vi "Digitizer_Trigger_Selection.vi"(3 "Error In":errorcluster, 4 "Channel Parameters In":T1, 5 "instrument handle in":refnum<k15>) -> (0 "error out":errorcluster, 1 "Channel Parameters Out":T1, 2 "instrument handle out":refnum<k15>)   [LabVIEW 2010]
uses:
  Typedef-Channel Parameters.ctl
  <instrlib>/niScope/Controls/niScope trigger slope.ctl
  <instrlib>/niScope/Controls/niScope trigger source.ctl
  <instrlib>/niScope/Controls/niScope export destinations.ctl
  <instrlib>/niScope/Controls/niScope exportable signals.ctl
  <instrlib>/niScope/Controls/niScope trigger source digital.ctl
  <instrlib>/niScope/Configure/Trigger/niScope Configure Trigger Edge.vi
  <instrlib>/niScope/Configure/Trigger/niScope Configure Trigger Digital.vi
  <instrlib>/niScope/Configure/Trigger/niScope Configure Trigger Immediate.vi
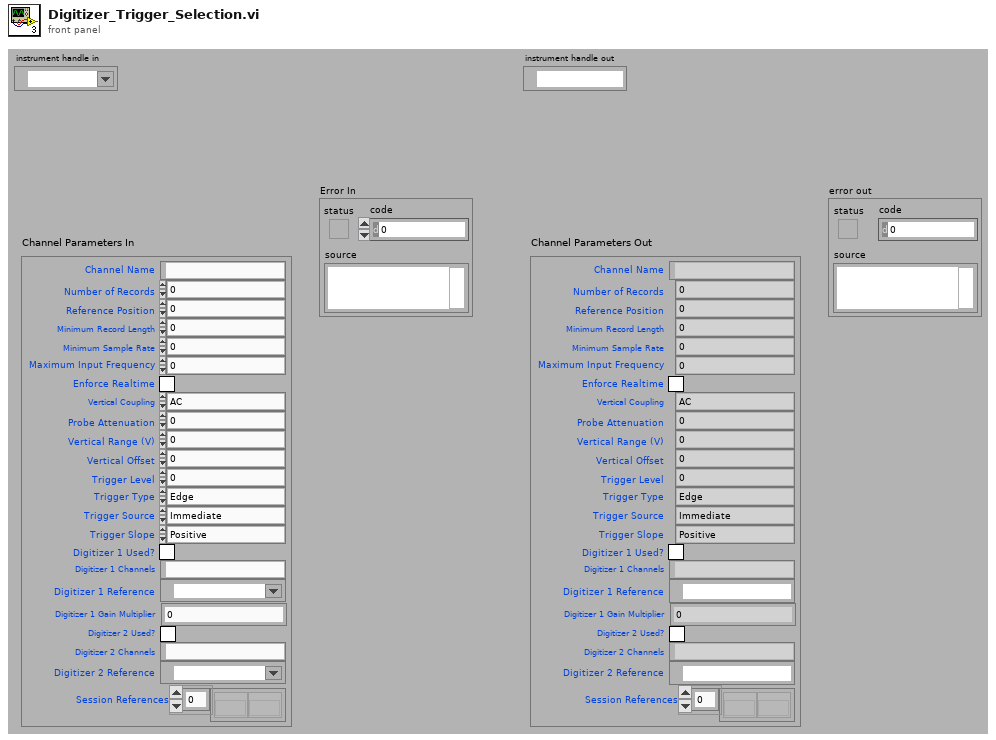
[diagram p1: front panel]
types:
  T1 = typedef "Typedef-Channel Parameters.ctl" = cluster{"Channel Name":string, "Number of Records":i32, "Reference Position":dbl, "Minimum Record Length":i32, "Minimum Sample Rate":dbl, "Maximum Input Frequency":dbl, "Enforce Realtime":bool, "Vertical Coupling":enum16{"AC", "DC", "Ground"}, "Probe Attenuation":dbl, "Vertical Range (V)":dbl, "Vertical Offset":dbl, "Trigger Level":dbl, "Trigger Type":enum16{"Edge", "Digital", "Immediate"}, "Trigger Source":enum16{"Immediate", "Channel 0", "Channel 1", "Channel 2", "Channel 3", "Channel 4", "Channel 5", "Channel 6", "Channel 7", "Extermal TRIG", "Software Trigger", "RTSI 0", "RTSI 1", "RTSI 2", "RTSI 3", "RTSI 4", "RTSI 5", "RTSI 6", "PF 0", "PF 1", "PF 2", "PXI Star Trigger"}, "Trigger Slope":enum16{"Positive", "Negative"}, "Digitizer 1 Used?":bool, "Digitizer 1 Channels":string, "Digitizer 1 Reference":refnum<k15>, "Digitizer 1 Gain Multiplier":dbl, "Digitizer 2 Used?":bool, "Digitizer 2 Channels":string, "Digitizer 2 Reference":refnum<k15>, "Session References":refnum<k20>[]}
  T2 = enum16{"Immediate", "Channel 0", "Channel 1", "Channel 2", "Channel 3", "Channel 4", "Channel 5", "Channel 6", "Channel 7", "Extermal TRIG", "Software Trigger", "RTSI 0", "RTSI 1", "RTSI 2", "RTSI 3", "RTSI 4", "RTSI 5", "RTSI 6", "PF 0", "PF 1", "PF 2", "PXI Star Trigger"}
  T3 = typedef "niScope trigger source.ctl" = string
  T4 = typedef "niScope export destinations.ctl" = string
  T5 = typedef "niScope trigger source digital.ctl" = string
  T6 = typedef "niScope trigger slope.ctl" = i32
  T7 = typedef "niScope exportable signals.ctl" = u16
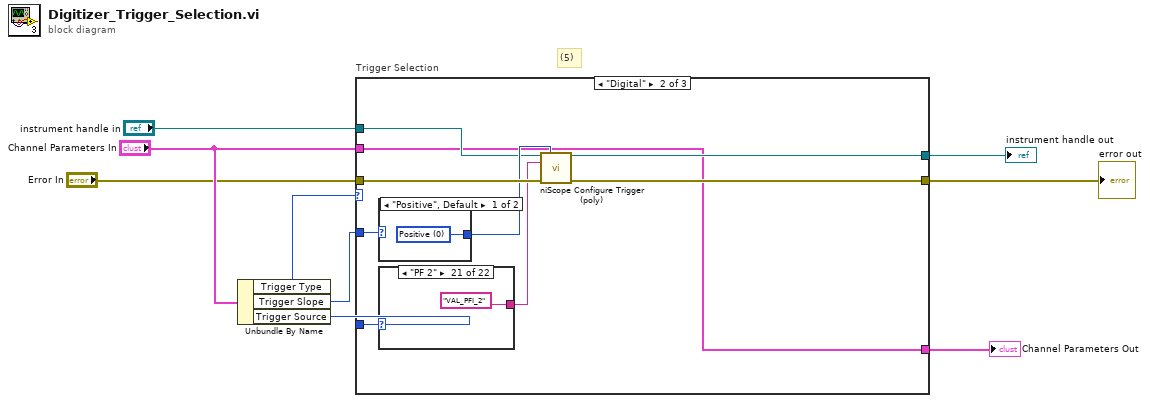
[diagram p0: block diagram]
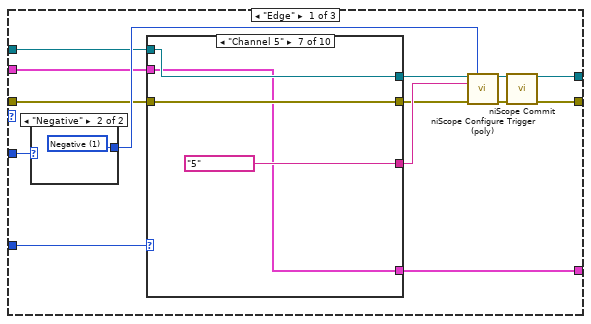
[diagram p2: hidden frame]
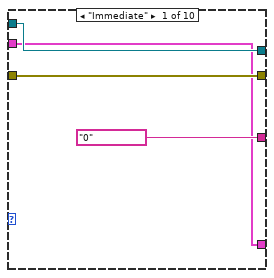
[diagram p3: hidden frame]
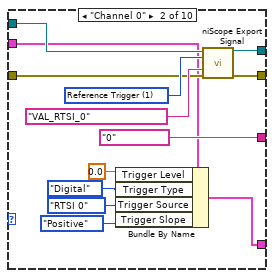
[diagram p4: hidden frame]
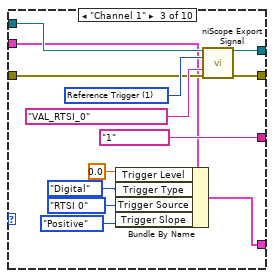
[diagram p5: hidden frame]
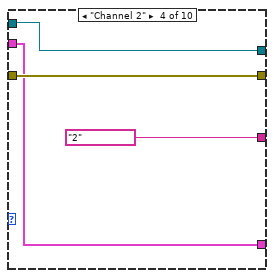
[diagram p6: hidden frame]
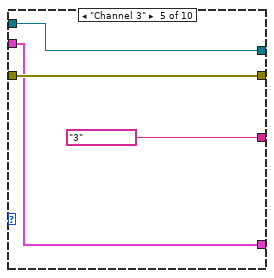
[diagram p7: hidden frame]
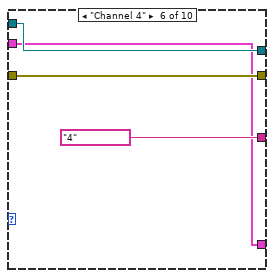
[diagram p8: hidden frame]
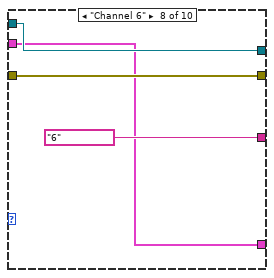
[diagram p9: hidden frame]
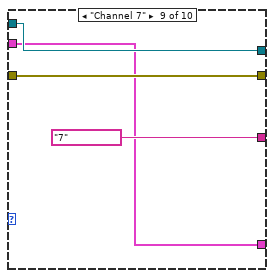
[diagram p10: hidden frame]
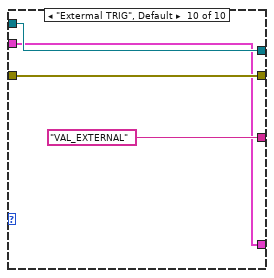
[diagram p11: hidden frame]
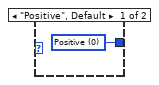
[diagram p12: hidden frame]
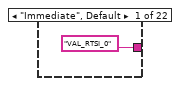
[diagram p13: hidden frame]
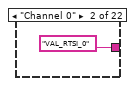
[diagram p14: hidden frame]
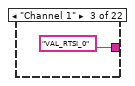
[diagram p15: hidden frame]
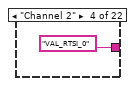
[diagram p16: hidden frame]
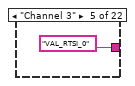
[diagram p17: hidden frame]
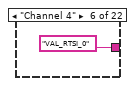
[diagram p18: hidden frame]
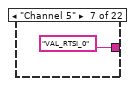
[diagram p19: hidden frame]
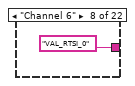
[diagram p20: hidden frame]
diagram:
  # "(5)"
  n1 = Unbundle By Name("Channel Parameters In") -> ("Trigger Type"=w1:enum16{"Edge", "Digital", "Immediate"}, "Trigger Slope"=w3:enum16{"Positive", "Negative"}, "Trigger Source"=w4:T2)
  n2 = case "Trigger Selection" shown="\"Digital\"" w1 {
    tunnel: "Error In" -> [w16 w92 w121]
    tunnel: [w18 w88 w120] -> w5
    tunnel: [w19 w89 w118] -> w9
    tunnel: w3 -> [w14 w87 _]
    tunnel: w4 -> [w13 w86 _]
    tunnel: [w12 w84 w117] -> w8
    tunnel: "Channel Parameters In" -> [w10 w84 w117]
    tunnel: "instrument handle in" -> [w11 w85 w119]
    frame "Edge" {
      n3 = case shown="\"Negative\"" w14 {
        tunnel: [w82 w83] -> w23
        frame "Positive", Default {
          w82 = T6 0 items=["Positive", "Negative"] ("trigger slope")
        }
        frame "Negative" {
          w83 = T6 1 items=["Positive", "Negative"] ("trigger slope")
        }
      }
      n4 = case shown="\"Channel 5\"" w13 {
        tunnel: [T3 "0" ("trigger source") T3 "0" ("trigger source") T3 "1" ("trigger source") T3 "2" ("trigger source") T3 "3" ("trigger source") T3 "4" ("trigger source") T3 "5" ("trigger source") T3 "6" ("trigger source") T3 "7" ("trigger source") T3 "VAL_EXTERNAL" ("trigger source")] -> w22
        tunnel: [w25 w36 w50 w55 w59 w63 w67 w71 w75 w79] -> w17
        tunnel: w16 -> [w26 w37 w49 w56 w60 w64 w68 w72 w76 w80]
        tunnel: [w26 w35 w48 w56 w60 w64 w68 w72 w76 w80] -> w15
        tunnel: [w24 w29 w43 w54 w58 w62 w66 w70 w74 w78] -> w12
        tunnel: w11 -> [w25 w30 w42 w55 w59 w63 w67 w71 w75 w79]
        tunnel: w10 -> [w24 w28 w41 w54 w58 w62 w66 w70 w74 w78]
        frame "Immediate" {
        }
        frame "Channel 0" {
          w38 = T7 1 items=["None"=0, "Start Trigger"=2, "Advance Trigger"=5, "Reference Trigger"=1, "End of Record Event"=4, "End of Acquisition Event"=3, "Ready for Start Event"=7, "Ready for Advance Event"=6, "Ready for Reference Event"=10, "Reference Clock"=100, "Sample Clock"=101, "5 Volt Power"=13] ("signal")
          n5 = Bundle By Name(cluster=w28, "Trigger Level"=0.0, "Trigger Type"=enum16{"Edge", "Digital", "Immediate"}."Digital", "Trigger Source"=T2."RTSI 0", "Trigger Slope"=enum16{"Positive", "Negative"}."Positive") -> (w29:T1)
          n6 = call <instrlib>:"niScope Export Signal.vi"("instrument handle"=w30, "signal"=w38, "output terminal"=T4 "VAL_RTSI_0", "error in"=w37) -> ("instrument handle out"=w36:refnum<k15>, "error out"=w35:errorcluster)  [unwired: 10 in]
        }
        frame "Channel 1" {
          w51 = T7 1 items=["None"=0, "Start Trigger"=2, "Advance Trigger"=5, "Reference Trigger"=1, "End of Record Event"=4, "End of Acquisition Event"=3, "Ready for Start Event"=7, "Ready for Advance Event"=6, "Ready for Reference Event"=10, "Reference Clock"=100, "Sample Clock"=101, "5 Volt Power"=13] ("signal")
          n7 = Bundle By Name(cluster=w41, "Trigger Level"=0.0, "Trigger Type"=enum16{"Edge", "Digital", "Immediate"}."Digital", "Trigger Source"=T2."RTSI 0", "Trigger Slope"=enum16{"Positive", "Negative"}."Positive") -> (w43:T1)
          n8 = call <instrlib>:"niScope Export Signal.vi"("instrument handle"=w42, "signal"=w51, "output terminal"=T4 "VAL_RTSI_0", "error in"=w49) -> ("instrument handle out"=w50:refnum<k15>, "error out"=w48:errorcluster)  [unwired: 10 in]
        }
        frame "Channel 2" {
        }
        frame "Channel 3" {
        }
        frame "Channel 4" {
        }
        frame "Channel 5" {
        }
        frame "Channel 6" {
        }
        frame "Channel 7" {
        }
        frame "Extermal TRIG", Default {
        }
      }
      n9 = call-poly <instrlib>:"niScope Configure Trigger (poly).vi"("instrument handle"=w17, "trigger slope"=w23, "trigger source"=w22, "error in"=w15) -> ("instrument handle out"=w21:refnum<k15>, "error out"=w20:errorcluster)  [unwired: 10 in]
      n10 = call <instrlib>:"niScope Commit.vi"("instrument handle"=w21, "error in"=w20) -> ("instrument handle out"=w19:refnum<k15>, "error out"=w18:errorcluster)  [unwired: 12 in]
    }
    frame "Digital" {
      n11 = case shown="\"Positive\", Default" w87 {
        tunnel: [w115 w116] -> w91
        frame "Positive", Default {
          w115 = T6 0 items=["Positive", "Negative"] ("trigger slope")
        }
        frame "Negative" {
          w116 = T6 1 items=["Positive", "Negative"] ("trigger slope")
        }
      }
      n12 = case shown="\"PF 2\"" w86 {
        tunnel: [T5 "VAL_RTSI_0" ("trigger source") T5 "VAL_RTSI_0" ("trigger source") T5 "VAL_RTSI_0" ("trigger source") T5 "VAL_RTSI_0" ("trigger source") T5 "VAL_RTSI_0" ("trigger source") T5 "VAL_RTSI_0" ("trigger source") T5 "VAL_RTSI_0" ("trigger source") T5 "VAL_RTSI_0" ("trigger source") T5 "VAL_RTSI_0" ("trigger source") T5 "VAL_RTSI_0" ("trigger source") T5 "VAL_RTSI_0" ("trigger source") T5 "VAL_RTSI_0" ("trigger source") T5 "VAL_RTSI_1" ("trigger source") T5 "VAL_RTSI_2" ("trigger source") T5 "VAL_RTSI_3" ("trigger source") T5 "VAL_RTSI_4" ("trigger source") T5 "VAL_RTSI_5" ("trigger source") T5 "VAL_RTSI_6" ("trigger source") T5 "VAL_PFI_0" ("trigger source") T5 "VAL_PFI_1" ("trigger source") T5 "VAL_PFI_2" ("trigger source") T5 "VAL_PXI_STAR" ("trigger source")] -> w90
        frame "Immediate", Default {
        }
        frame "Channel 0" {
        }
        frame "Channel 1" {
        }
        frame "Channel 2" {
        }
        frame "Channel 3" {
        }
        frame "Channel 4" {
        }
        frame "Channel 5" {
        }
        frame "Channel 6" {
        }
        frame "Channel 7" {
        }
        frame "Extermal TRIG" {
        }
        frame "Software Trigger" {
        }
        frame "RTSI 0" {
        }
        frame "RTSI 1" {
        }
        frame "RTSI 2" {
        }
        frame "RTSI 3" {
        }
        frame "RTSI 4" {
        }
        frame "RTSI 5" {
        }
        frame "RTSI 6" {
        }
        frame "PF 0" {
        }
        frame "PF 1" {
        }
        frame "PF 2" {
        }
        frame "PXI Star Trigger" {
        }
      }
      n13 = call-poly <instrlib>:"niScope Configure Trigger (poly).vi"("instrument handle"=w85, "trigger slope"=w91, "trigger source"=w90, "error in"=w92) -> ("instrument handle out"=w89:refnum<k15>, "error out"=w88:errorcluster)  [unwired: 10 in]
    }
    frame "Immediate", Default {
      n14 = call-poly <instrlib>:"niScope Configure Trigger (poly).vi"("instrument handle"=w119, "error in"=w121) -> ("instrument handle out"=w118:refnum<k15>, "error out"=w120:errorcluster)  [unwired: 12 in]
    }
  }
  "instrument handle out" <- w9
  "Channel Parameters Out" <- w8
  "error out" <- w5
